vi "get update file.vi"(11 "服务器信息":T1={"host"="27.154.58.30", "port"=8020, "user"="std", "password"="std23506", "远端地址"="/微站/室外总磷总氮高压过滤无主板新电路板/一体化微型水质监测站.exe"}) -> ()   [LabVIEW 2016, in "update.lvlib"]
uses:
  update.lvlib
  <vilib>/Utility/error.llb/DialogType.ctl
  <vilib>/httpClient/POSTBuffer.vi
  <vilib>/regexp/Match Regular Expression.xnode
  <vilib>/httpClient/LabVIEWHTTPClient.lvlib
panel:
  out "文件大小":i32
  out "headers":string caption="头部"
  out "滑动杆":dbl(slide) scale=0.0..100.0
  out "大小":i64
  out "command":string caption="命令"
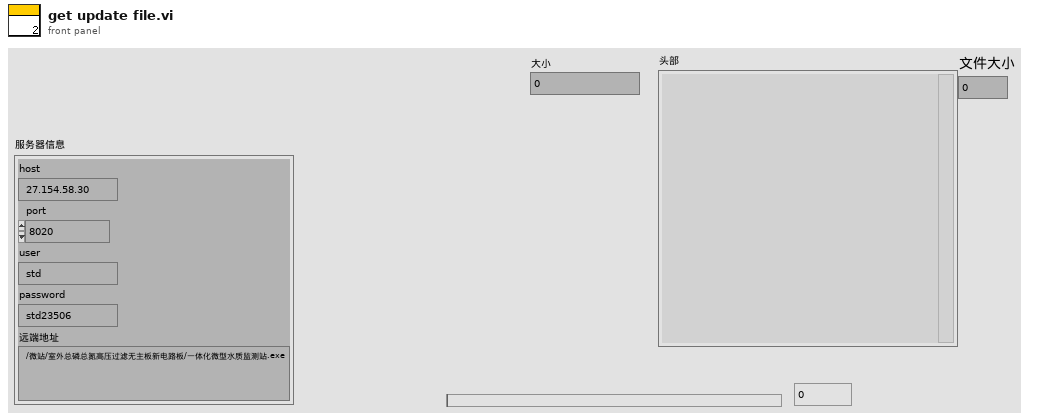
[diagram p1: front panel]
types:
  T1 = cluster{"host":string, "port":u16, "user":string, "password":string, "远端地址":string}
  T2 = cluster{"command":string, "last status string":string, dbl}
  T3 = cluster{"command":string, "last status string":string, "process":dbl}
  T4 = enum16{"open", "replace", "create", "open or create", "replace or create", "replace or create with confirmation"}
  T5 = typedef "LabVIEWHTTPClient.lvlib/ClientHandle.ctl" = refnum<k1>
  T6 = typedef "DialogType.ctl" = u16
  T7 = enum32{"invalid app kind", "Development System", "Run Time System", "Student Edition", "Embedded LabVIEW", "Evaluation", "Custom"}
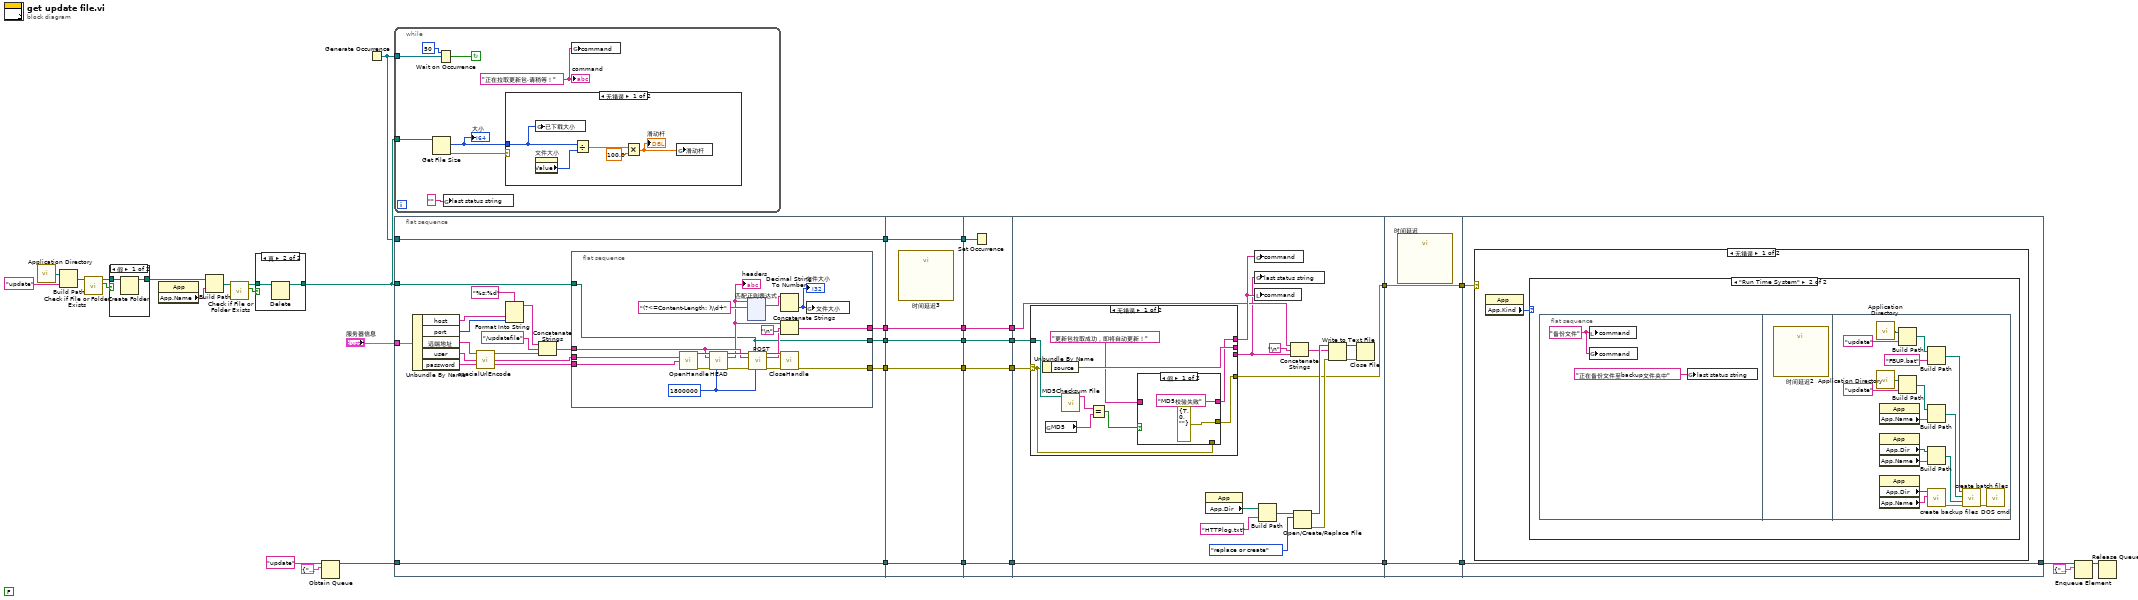
[diagram p0: block diagram]
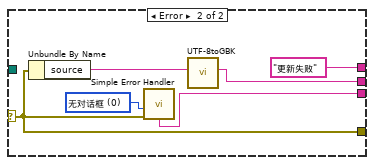
[diagram p6: hidden frame]
diagram:
  (unwired) FALSE ("FTP链接结束")
  n1 = call <vilib>:"Application Directory.vi"() -> ("Application Directory"=w29:path)
  n2 = Build Path(base path=w29, name or relative path="update" ("名称或相对路径")) -> (appended path=w30:path)
  n3 = call <vilib>:"Check if File or Folder Exists.vi"("path"=w30) -> ("file or folder exists?"=w31:bool, "dup path"=w32:path)  [unwired: 8 in, 1 out]
  n4 = case shown="假" w31 {
    tunnel: w32 -> [w39 w40]
    tunnel: [w38 w40] -> w27
    frame False {
      n5 = Create Folder(path (use dialog)=w39) -> (created path=w38:path)  [unwired: 2 in, 2 out]
    }
    frame True {
    }
  }
  n6 = property class="App"() -> ("App.Name"=w15:string)  [unwired: 2 in, 2 out]
  n7 = Build Path(base path=w27, name or relative path=w15) -> (appended path=w26:path)
  n8 = call <vilib>:"Check if File or Folder Exists.vi"("path"=w26) -> ("file or folder exists?"=w25:bool, "dup path"=w24:path)  [unwired: 8 in, 1 out]
  n9 = case shown="真" w25 {
    tunnel: w24 -> [w41 w43]
    tunnel: [w41 w42] -> w22
    frame False {
    }
    frame True {
      n10 = Delete(path (use dialog)=w43) -> (deleted path=w42:path)  [unwired: 4 in, 2 out]
    }
  }
  n11 = Obtain Queue(name (unnamed)="update" ("名称（未命名）"), element data type=T3 {"command"="", "last status string"="", "process"=0.0}) -> (queue out=w23:refnum<queue>)  [unwired: 3 in, 2 out]
  n12 = Generate Occurrence() -> (w13:refnum<k4>)
  n13 = while {
    tunnel: w22 -> [w51]
    tunnel: w13 -> [w48]
    stop <- w46 continue-if-true
    w45 = "正在拉取更新包,请稍等！" ("格式字符串")
    n14 = Get File Size(file=w51) -> (size (in bytes)=w49:i64, 0:w50:errorcluster)  [unwired: 1 in, 1 out]
    "大小" <- w49
    n15 = Wait on Occurrence(2:w48, 3:50 ("毫秒超时(-1)")) -> (0:w46:bool)  [unwired: 1 in]
    n16 = global write "更新全局变量.vi" "last status string"("" ("last status string")) -> ()
    n17 = case shown="无错误" w50 {
      tunnel: w49 -> [w55 _]
      frame No Error {
        n18 = global write "更新全局变量.vi" "已下载大小"(w55) -> ()
        n19 = property on="文件大小" class="DigNum (严格)"() -> ("Value"=w53:i32)  [unwired: 2 in, 2 out]
        n20 = Divide(x=w55, y=w53) -> (x/y=w56:dbl)
        n21 = Multiply(x=w56, y=100.0) -> (x*y=w54:dbl)
        "滑动杆" <- w54
        n22 = global write "更新全局变量.vi" "滑动杆"(w54) -> ()
      }
      frame Error {
      }
    }
    n23 = global write "更新全局变量.vi" "command"(w45) -> ()
    "command" <- w45
  }
  n24 = flat-sequence {
    tunnel: [w59] -> w21
    tunnel: w23 -> [w73]
    tunnel: [w73] -> w20
    tunnel: w22 -> [w60]
    tunnel: "服务器信息" -> [w65]
    tunnel: w13 -> [w72]
    tunnel: [w72] -> w12
    tunnel: [w58] -> w4
    tunnel: [w57] -> w1
    tunnel: w21 -> [w211]
    tunnel: [w211] -> w11
    tunnel: w20 -> [w210]
    tunnel: [w210] -> w9
    tunnel: w12 -> [w209]
    tunnel: [w209] -> w7
    tunnel: [w208] -> w5
    tunnel: w4 -> [w208]
    tunnel: [w207] -> w2
    tunnel: w1 -> [w207]
    tunnel: w11 -> [w216]
    tunnel: [w216] -> w10
    tunnel: w9 -> [w215]
    tunnel: [w215] -> w8
    tunnel: w7 -> [w214]
    tunnel: [w213] -> w6
    tunnel: w5 -> [w213]
    tunnel: [w212] -> w3
    tunnel: w2 -> [w212]
    tunnel: w10 -> [w233]
    tunnel: [w218] -> w19
    tunnel: w8 -> [w231]
    tunnel: [w231] -> w17
    tunnel: w6 -> [w222]
    tunnel: w3 -> [w217]
    tunnel: w19 -> [w254]
    tunnel: [w254] -> w18
    tunnel: w17 -> [w253]
    tunnel: [w253] -> w16
    tunnel: w18 -> [w255]
    tunnel: w16 -> [w256]
    tunnel: [w256] -> w35
    frame #0 {
      n25 = Unbundle By Name(w65) -> ("host"=w69:string, "port"=w68:u16, "远端地址"=w64:string, "user"=w63:string, "password"=w62:string)
      n26 = call "specialUrlEncode.vi"("str"=w64) -> ("UrlEncode"=w70:string)  [unwired: 10 in]
      n27 = Format Into String(format string="%s:%d" ("格式字符串"), w69, w68) -> (resulting string=w67:string)  [unwired: 2 in, 1 out]
      n28 = Concatenate Strings(w67, "/updatefile", w70) -> (w61:string)
      n29 = flat-sequence {
        tunnel: w63 -> [w92]
        tunnel: w62 -> [w91]
        tunnel: w61 -> [w77]
        tunnel: w60 -> [w74]
        tunnel: [w87] -> w59
        tunnel: [w85] -> w58
        tunnel: [w74] -> w57
        frame #0 {
          w75 = 1800000 ("timeout (10000)")
          n30 = call <vilib>:"OpenHandle.vi"("username"=w92, "password"=w91) -> ("client handle out"=w81:T5, "error out"=w79:errorcluster)  [unwired: 12 in]
          n31 = call <vilib>:"HEAD.vi"("client handle"=w81, "url"=w77, "error in (no error)"=w79, "timeout (10000)"=w75) -> ("client handle out"=w80:T5, "headers"=w76:string, "error out"=w78:errorcluster)  [unwired: 9 in]
          "headers" <- w76
          n32 = xnode "匹配正则表达式"("输入字符串"=w76, "正则表达式"="(?<=Content-Length: )\\d+") -> ("所有匹配"=w89:string)  [unwired: 4 in, 4 out]
          n33 = call-poly <vilib>:"POST.vi"("client handle"=w80, "output file"=w74, "url"=w77, "error in (no error)"=w78, "timeout (10000)"=w75) -> ("client handle out"=w84:T5, "headers"=w82:string, "error out"=w83:errorcluster)  [unwired: 7 in, 1 out]
          n34 = Decimal String To Number(string=w89) -> (number=w88:i32)  [unwired: 2 in, 1 out]
          "文件大小" <- w88
          n35 = Concatenate Strings(w76, "\n", w82) -> (w85:string)
          n36 = call <vilib>:"CloseHandle.vi"("client handle"=w84, "error in (no error)"=w83) -> ("error out"=w87:errorcluster)  [unwired: 13 in]
          n37 = global write "更新全局变量.vi" "文件大小"(w88) -> ()
        }
      }
    }
    frame #1 {
      n38 = call "时间延迟3"() -> ()  [unwired: 11 in, 1 out]
    }
    frame #2 {
      n39 = Set Occurrence(w214) -> ()
    }
    frame #3 {
      n40 = case shown="无错误" w233 {
        selector: w233 -> [w234 w247]
        tunnel: [w236 "更新失败" ("command")] -> w232
        tunnel: [w242 w250] -> _
        tunnel: [_ w248] -> w219
        tunnel: [w235 w247] -> w218
        tunnel: w217 -> [w241 _]
        frame No Error {
          n41 = Unbundle By Name(w234) -> ("source"=w242:string)
          n42 = global read "更新全局变量.vi" "MD5"() -> (w239:string)
          n43 = call <vilib>:"MD5Checksum File.vi"("Path"=w241) -> ("MD5 message-digest"=w240:string)  [unwired: 9 in, 1 out]
          n44 = Equal?(x=w240, y=w239) -> (x = y?=w238:bool)
          n45 = case shown="假" w238 {
            tunnel: ["MD5校验失败" w246] -> w236
            tunnel: "更新包拉取成功，即将自动更新！" ("command") -> [_ w246]
            tunnel: [errorcluster {"status"=TRUE, "code"=0, "source"=""} ("error IO") w245] -> w235
            tunnel: w234 -> [_ w245]
            frame False {
            }
            frame True {
              # "MD5相等"
            }
          }
        }
        frame Error {
          w249 = T6 0 items=["无对话框", "确定信息", "继续或停止信息", "确定信息＋警告", "继续/停止+警告"] ("type of dialog (OK msg:1)")
          n46 = Unbundle By Name(w247) -> ("source"=w251:string)
          n47 = call <vilib>:"Simple Error Handler.vi"("type of dialog (OK msg:1)"=w249, "error in (no error)"=w247) -> ("message"=w248:string)  [unwired: 3 in, 4 out]
          n48 = call "UTF-8toGBK.vi"("UTF-8"=w251) -> ("GBK"=w250:string)  [unwired: 9 in, 1 out]
        }
      }
      n49 = property class="App"() -> ("App.Dir"=w224:path)  [unwired: 2 in, 2 out]
      n50 = global write "更新全局变量.vi" "command"(w232) -> ()
      n51 = global write "更新全局变量.vi" "last status string"(w219) -> ()
      n52 = local write "command"(w232) -> ()
      n53 = Build Path(base path=w224, name or relative path="HTTPlog.txt" ("名称或相对路径")) -> (appended path=w226:path)
      n54 = Concatenate Strings(w222, "\n", w219) -> (w220:string)
      n55 = Open/Create/Replace File(file path (use dialog)=w226, operation (0:open)=T4."replace or create" ("操作(0:open)")) -> (refnum out=w229:refnum<file>, error out=w228:errorcluster)  [unwired: 4 in, 1 out]
      n56 = Write to Text File(file (use dialog)=w229, text=w220, error in=w228) -> (refnum out=w230:refnum<file>, error out=w223:errorcluster)  [unwired: 1 in, 1 out]
      n57 = Close File(refnum=w230, error in=w223) -> ()  [unwired: 2 out]
    }
    frame #4 {
      n58 = call "时间延迟"() -> ()  [unwired: 11 in, 1 out]
    }
    frame #5 {
      n59 = case shown="无错误" w255 {
        frame No Error {
          n60 = property class="App"() -> ("App.Kind"=w257:T7)  [unwired: 2 in, 2 out]
          n61 = case shown="\"Run Time System\"" w257 {
            frame "invalid app kind", Default {
            }
            frame "Run Time System" {
              n62 = flat-sequence {
                frame #0 {
                  w259 = "备份文件" ("command")
                  n63 = local write "command"(w259) -> ()
                  n64 = global write "更新全局变量.vi" "command"(w259) -> ()
                  n65 = global write "更新全局变量.vi" "last status string"("正在备份文件至backup文件夹中" ("last status string")) -> ()
                }
                frame #1 {
                  n66 = call "时间延迟2"() -> ()  [unwired: 11 in, 1 out]
                }
                frame #2 {
                  n67 = call <vilib>:"Application Directory.vi"() -> ("Application Directory"=w262:path)
                  n68 = call <vilib>:"Application Directory.vi"() -> ("Application Directory"=w272:path)
                  n69 = property class="App"() -> ("App.Name"=w269:string)  [unwired: 2 in, 2 out]
                  n70 = property class="App"() -> ("App.Dir"=w268:path, "App.Name"=w267:string)  [unwired: 2 in, 2 out]
                  n71 = property class="App"() -> ("App.Dir"=w266:path, "App.Name"=w265:string)  [unwired: 2 in, 2 out]
                  n72 = Build Path(base path=w262, name or relative path="update" ("名称或相对路径")) -> (appended path=w263:path)
                  n73 = Build Path(base path=w272, name or relative path="update" ("名称或相对路径")) -> (appended path=w270:path)
                  n74 = Build Path(base path=w263, name or relative path="FBUP.bat" ("batch file name")) -> (appended path=w274:path)
                  n75 = Build Path(base path=w270, name or relative path=w269) -> (appended path=w261:path)
                  n76 = Build Path(base path=w268, name or relative path=w267) -> (appended path=w260:path)
                  n77 = call "create backup files.vi"("execute file name"=w265, "路径"=w266) -> ("error out"=w275:errorcluster)  [unwired: 9 in]
                  n78 = call "create batch files.vi"("错误输入（无错误）"=w275, "Targe Path"=w260, "Source Path"=w261, "Batch file"=w274) -> ("错误输出"=w276:errorcluster)  [unwired: 7 in]
                  n79 = call "DOS cmd.vi"("错误输入（无错误）"=w276) -> ()  [unwired: 10 in, 1 out]
                }
              }
            }
          }
        }
        frame Error {
        }
      }
    }
  }
  n80 = Enqueue Element(queue=w35, element=T2 {"command"="stop", "last status string"="", 0.0} ("元素")) -> (queue out=w34:refnum<queue>)  [unwired: 2 in, 2 out]
  n81 = Release Queue(queue=w34) -> ()  [unwired: 2 in, 3 out]
